vi "get stable RF voltage.vi"(9 "diode steady state voltage":dbl, 10 "polarimeter task in":refnum<k21>, 11 "rf gen task in":refnum<k21>) -> (1 "stable voltage":dbl, 2 "polarimeter task out":refnum<k21>, 3 "rf gen task out":refnum<k21>)   [LabVIEW 2018]
uses:
  <vilib>/DAQmx/write.llb/DAQmx Write (Analog DBL 1Chan 1Samp).vi
  4f967cfa-f295-4c21-8527-c71cc98837c5.vi
  f9da4950-4a72-4538-adda-a8c4b27a076f.vi
  <vilib>/DAQmx/read.llb/DAQmx Read (Analog DBL 1Chan 1Samp).vi
  <vilib>/DAQmx/miscellaneous.llb/DAQmx Fill In Error Info.vi
panel:
  in  "start voltage":dbl=0.3 format="%#_13g"
  out "Waveform Chart":dbl(graph)
  out "current rf voltage in":dbl
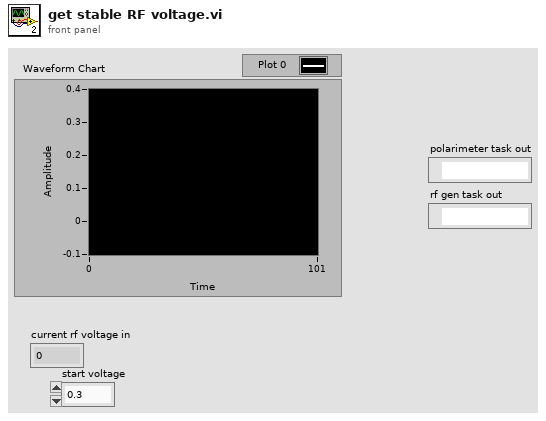
[diagram p1: front panel]
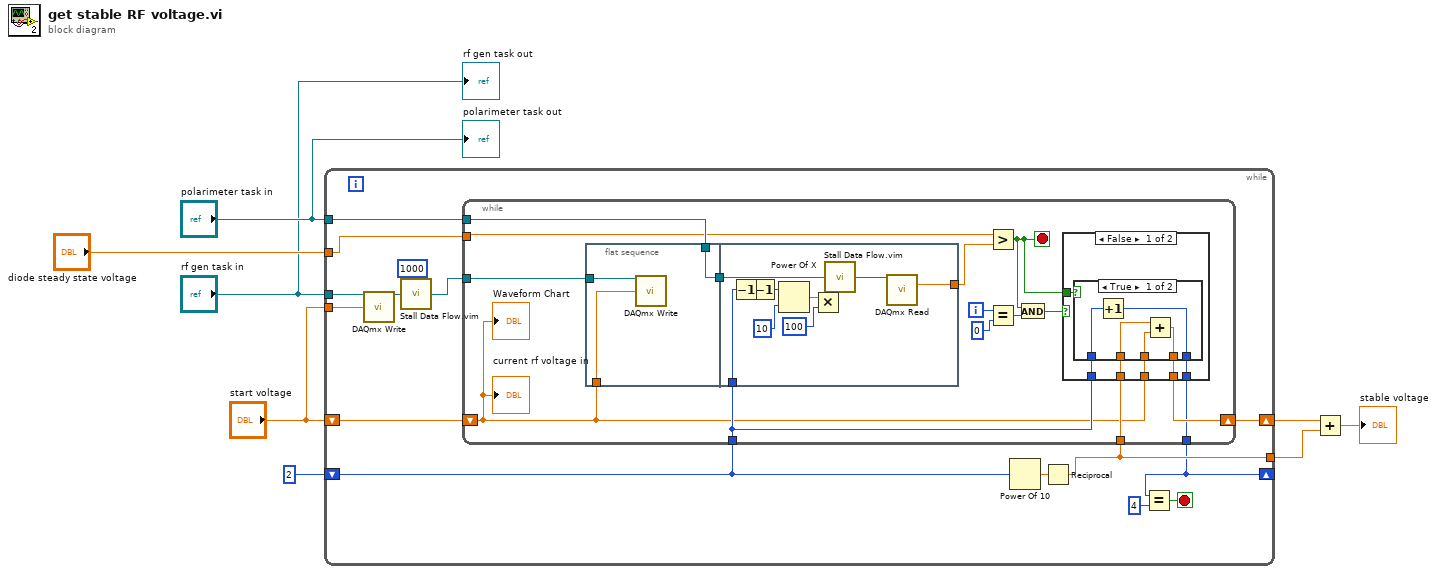
[diagram p0: block diagram]
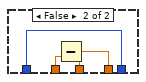
[diagram p2: hidden frame]
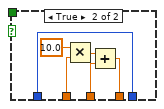
[diagram p3: hidden frame]
diagram:
  n1 = while {
    tunnel: "polarimeter task in" -> [w12]
    shift-right: [w16] -> w4
    shift-left: "start voltage" -> [w9]
    tunnel: "rf gen task in" -> [w20]
    tunnel: "start voltage" -> [w19]
    shift-right: [w13] -> _
    shift-left: 2 -> [w15]
    tunnel: [w14] -> w6
    tunnel: "diode steady state voltage" -> [w10]
    stop <- w17 stop-if-true
    n2 = call-poly <vilib>:"DAQmx Write.vi"("task/channels in"=w20, "data"=w19) -> ("task out"=w22:refnum<k21>)  [unwired: 11 in, 2 out]
    n3 = call "Stall Data Flow.vim"("value in"=w22, "milliseconds to wait"=u32 1000) -> ("value out"=w11:refnum<k21>)  [unwired: 1 out]
    n4 = Power Of 10(x=w15) -> (10^x=w23:dbl)
    n5 = Reciprocal(x=w23) -> (1/x=w14:dbl)
    n6 = while {
      tunnel: w12 -> [w30]
      tunnel: w11 -> [w31]
      shift-right: [w33] -> w16
      shift-left: w9 -> [w25]
      tunnel: w14 -> [w34]
      tunnel: w15 -> [w28]
      tunnel: [w32] -> w13
      tunnel: w10 -> [w24]
      i -> [w38]
      stop <- w26 stop-if-true
      n7 = flat-sequence {
        tunnel: w25 -> [w41]
        tunnel: w31 -> [w40]
        tunnel: w30 -> [w39]
        tunnel: [w39] -> w29
        tunnel: w29 -> [w44]
        tunnel: w28 -> [w43]
        tunnel: [w42] -> w27
        frame #0 {
          n8 = call-poly <vilib>:"DAQmx Write.vi"("task/channels in"=w40, "data"=w41) -> ()  [unwired: 11 in, 3 out]
        }
        frame #1 {
          n9 = Decrement(x=w43) -> (x-1=w49:i32)
          n10 = Decrement(x=w49) -> (x-1=w45:i32)
          n11 = Power Of X(1:10 ("y"), 2:w45) -> (0:w46:dbl)
          n12 = Multiply(x=w46, y=100) -> (x*y=w47:dbl)
          n13 = call "Stall Data Flow.vim"("value in"=w44, "milliseconds to wait"=w47) -> ("value out"=w51:refnum<k21>)  [unwired: 1 out]
          n14 = call-poly <vilib>:"DAQmx Read.vi"("task/channels in"=w51) -> ("data"=w42:dbl)  [unwired: 12 in, 2 out]
        }
      }
      n15 = Greater?(x=w24, y=w27) -> (0:w26:bool)
      n16 = Equal?(x=w38, y=0) -> (x = y?=w36:bool)
      n17 = And(x=w26, y=w36) -> (x .and. y?=w35:bool)
      n18 = case shown="False" w35 {
        tunnel: w34 -> [w55 w72]
        tunnel: w25 -> [w56 w69]
        tunnel: [w57 w68] -> w33
        tunnel: w28 -> [w54 w67]
        tunnel: [w53 w67] -> w32
        tunnel: w26 -> [w52 _]
        frame False {
          n19 = case shown="True" w52 {
            tunnel: [w62 w64] -> w57
            tunnel: w56 -> [w61 w66]
            tunnel: w55 -> [w60 w65]
            tunnel: w54 -> [w59 w63]
            tunnel: [w58 w63] -> w53
            frame True {
              n20 = Increment(x=w59) -> (x+1=w58:i32)
              n21 = Add(x=w60, y=w61) -> (x+y=w62:dbl)
            }
            frame False {
              n22 = Subtract(x=w66, y=w65) -> (x-y=w64:dbl)
            }
          }
        }
        frame True {
          n23 = Multiply(x=10.0, y=w72) -> (x*y=w70:dbl)
          n24 = Add(x=w70, y=w69) -> (x+y=w68:dbl)
        }
      }
      "Waveform Chart" <- w25
      "current rf voltage in" <- w25
    }
    n25 = Equal?(x=w13, y=4) -> (x = y?=w17:bool)
  }
  n26 = Add(x=w4, y=w6) -> (x+y=→"stable voltage":dbl)
  "rf gen task out" <- "rf gen task in"
  "polarimeter task out" <- "polarimeter task in"
